vi "字符头匹配.vi"(10 "匹配字符数组":string[](array[string]), 11 "字符头":string) -> (2 "匹配结果":bool, 3 "匹配之后":string)   [LabVIEW 2016]
uses:
  <vilib>/regexp/Match Regular Expression.xnode
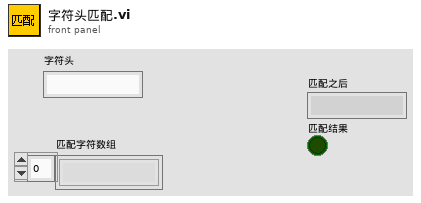
[diagram p1: front panel]
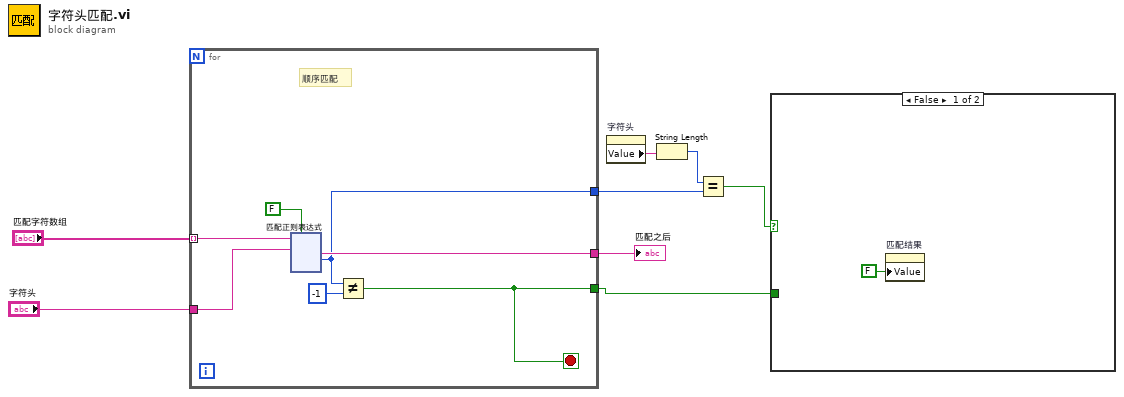
[diagram p0: block diagram]
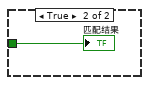
[diagram p2: hidden frame]
diagram:
  n1 = for {
    tunnel: "匹配字符数组" -> [w15] mode=indexing
    tunnel: "字符头" -> [w14]
    tunnel: [w11] -> w6
    tunnel: [w10] -> w1
    tunnel: [w9] -> w3
    stop <- w10 stop-if-true
    # "顺序匹配"
    n2 = xnode "匹配正则表达式"("input string"=w15, "regular expression"=w14, "ignore case? (F)"=FALSE ("忽略大小写？(F)")) -> ("after match"=w11:string, "offset past match"=w9:i32)  [unwired: 3 in, 3 out]
    n3 = Not Equal?(x=w9, y=-1) -> (x != y?=w10:bool)
  }
  "匹配之后" <- w6
  n4 = property on="字符头" class="Str"() -> ("Value"=w5:string)  [unwired: 2 in, 2 out]
  n5 = String Length(string=w5) -> (length=w4:i32)
  n6 = Equal?(x=w4, y=w3) -> (x = y?=w2:bool)
  n7 = case shown="False" w2 {
    tunnel: w1 -> [_ w131]
    frame False {
      n8 = property on="匹配结果" class="Bool (strict)"("Value"=FALSE ("匹配结果")) -> ()  [unwired: 2 in, 2 out]
    }
    frame True {
      "匹配结果" <- w131
    }
  }
